vi "ShowWindowGreyscale.vi"(8 "error in (no error)":errorcluster, 10 "Window Name":string, 11 "Greyscale Image":refnum<data-value>) -> (0 "error out":errorcluster, 3 "Greyscale Image (duplicate)":refnum<data-value>)   [LabVIEW 2020, in "g_ar_toolkit.image.lvlib"]
uses:
  g_ar_toolkit.image.lvlib
  <vilib>/Utility/error.llb/Error Cluster From Error Code.vi
  9022224c-4441-4334-9f82-39df2e645c64.vi
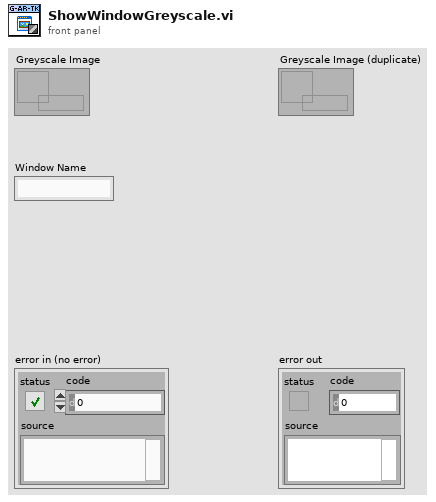
[diagram p1: front panel]
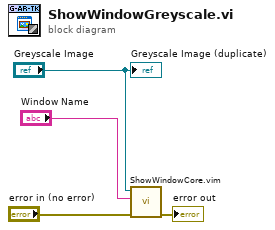
[diagram p0: block diagram]
diagram:
  n1 = call "ShowWindowCore.vim"("error in (no error)"="error in (no error)", "Window Name"="Window Name", "Img"="Greyscale Image") -> ("error out"=→"error out":errorcluster)  [unwired: 8 in]
  "Greyscale Image (duplicate)" <- "Greyscale Image"
